vi "Initialize_IMU_Interrupt.vi"(0 "dmp_sample_rate":i32=100, 5 "orientation":u32(ring)=112 items=["ORIENTATION_Z_UP"=136, "ORIENTATION_Z_DOWN"=396, "ORIENTATION_X_UP"=14, "ORIENTATION_X_DOWN"=266, "ORIENTATION_Y_UP"=112, "ORIENTATION_Y_DOWN"=336, "ORIENTATION_X_FORWARD"=133, "ORIENTATION_X_BACK"=161], 7 "enable_magnetometer":i32, 9 "dmp_interrupt_priority":i32=20 min=1 max=99 step=1, 11 "error in (no error)":errorcluster) -> (4 "IMU Event":refnum<user-event>, 6 "Event Registration Refnum":refnum<event-registration>, 10 "IMU Data":T1, 15 "error out":errorcluster)   [LabVIEW 2014]
uses:
  rc_interrupt/LV/Interrupt.lvlib
  <userlib>/UCSD Robotics Lab/Robotics-Cape/LV/libroboticscape.lvlib
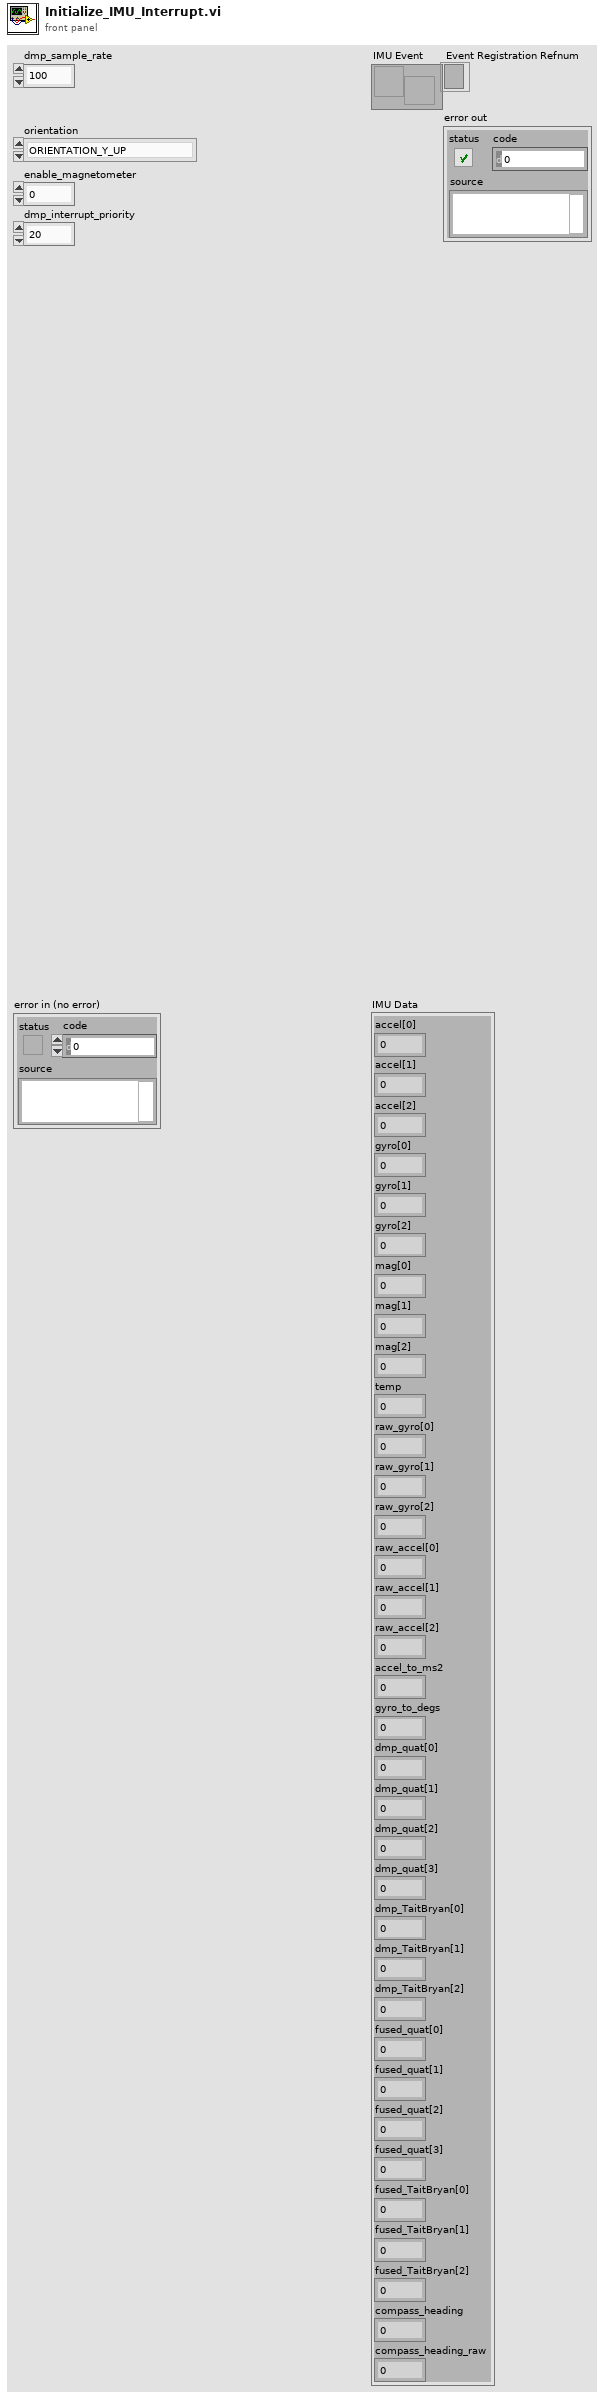
[diagram p1: front panel]
types:
  T1 = cluster{"accel[0]":sgl, "accel[1]":sgl, "accel[2]":sgl, "gyro[0]":sgl, "gyro[1]":sgl, "gyro[2]":sgl, "mag[0]":sgl, "mag[1]":sgl, "mag[2]":sgl, "temp":sgl, "raw_gyro[0]":i16, "raw_gyro[1]":i16, "raw_gyro[2]":i16, "raw_accel[0]":i16, "raw_accel[1]":i16, "raw_accel[2]":i16, "accel_to_ms2":sgl, "gyro_to_degs":sgl, "dmp_quat[0]":sgl, "dmp_quat[1]":sgl, "dmp_quat[2]":sgl, "dmp_quat[3]":sgl, "dmp_TaitBryan[0]":sgl, "dmp_TaitBryan[1]":sgl, "dmp_TaitBryan[2]":sgl, "fused_quat[0]":sgl, "fused_quat[1]":sgl, "fused_quat[2]":sgl, "fused_quat[3]":sgl, "fused_TaitBryan[0]":sgl, "fused_TaitBryan[1]":sgl, "fused_TaitBryan[2]":sgl, "compass_heading":sgl, "compass_heading_raw":sgl}
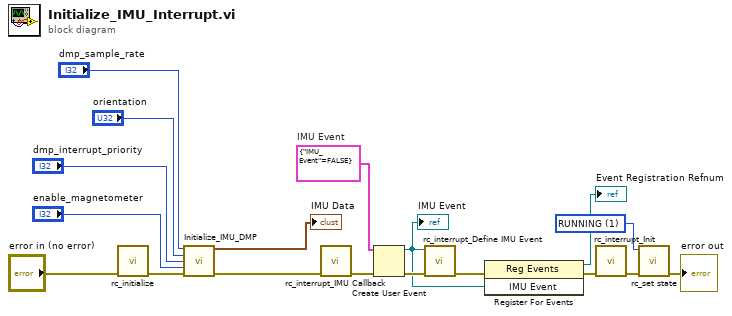
[diagram p0: block diagram]
diagram:
  w4 = u32 1 items=["UNINITIALIZED", "RUNNING", "PAUSED", "EXITING"] ("new_state")
  w17 = cluster{"IMU_Event":bool} {"IMU_Event"=FALSE}  # IMU Event
  n1 = call <userlib>:"rc_initialize.vi"("error in (no error)"="error in (no error)") -> ("error out"=w15:errorcluster)  [unwired: 9 in, 1 out]
  n2 = call "Initialize_IMU_DMP.vi"("dmp_sample_rate"="dmp_sample_rate", "orientation"="orientation", "dmp_interrupt_priority"="dmp_interrupt_priority", "enable_magnetometer"="enable_magnetometer", "error in (no error)"=w15) -> ("Data Out"=→"IMU Data":T1, "error out"=w14:errorcluster)  [unwired: 9 in]
  n3 = call "rc_interrupt_IMU Callback.vi"("error in (no error)"=w14) -> ("error out"=w13:errorcluster)  [unwired: 9 in, 1 out]
  n4 = Create User Event(user event datatype=w17, error in=w13) -> (user event=w10:refnum<user-event>, error out=w12:errorcluster)
  "IMU Event" <- w10
  n5 = call "rc_interrupt_Define IMU Event.vi"("error in (no error)"=w12, "user event in"=w10) -> ("error out"=w11:errorcluster)  [unwired: 8 in, 1 out]
  n6 = register-events(error in=w11, w10) -> (reference out=→"Event Registration Refnum":refnum<event-registration>, error out=w9:errorcluster)  [unwired: 1 in]
  n7 = call "rc_interrupt_Init.vi"("error in (no error)"=w9) -> ("error out"=w6:errorcluster)  [unwired: 9 in, 1 out]
  n8 = call <userlib>:"rc_set state.vi"("error in (no error)"=w6, "new_state"=w4) -> ("error out"=→"error out":errorcluster)  [unwired: 8 in, 1 out]
